vi "Main.vi"() -> ()   [LabVIEW 2020]
doc: "This template is for the Queued Message Handler design pattern.\n\nThe Event Handling Loop generates messages based on user interface actions.\n\nThe Message Handling Loop processes messages generated by the Event Handling Loop, or by other messages. The messages are string values, so new messages can be added easily to the Message Cases case structure in the Message Handling Loop. Each message cluster can also provide an optional value for Message Data, which is a variant that can be converted to whatever message-specific data is required."
uses:
  controls/UI Data.ctl
  support/Message Queue/Enqueue Message (Single).vi
  Global 1.vi
  <vilib>/Utility/error.llb/Error Cluster From Error Code.vi
  <vilib>/ErrorRing/Error Ring.xnode
  support/Message Queue/Message Queue.lvlib
  support/User Event - Stop/User Event - Stop.lvlib
panel:
  in  "Preferences":bool
  in  "Tab Control":enum32{"Main", "New Scenario", "Run Scenario"}(tab)
  in  "New Scenario":bool
  in  "Run Scenario":bool
  in  "Return":bool
  in  "Quit":bool
  in  "Edit Scenario":bool
  in  "Play Button":bool
  in  "Media Stop Button":bool
  out "number (0 to 1)":dbl
  out "Display <Replace Me>":string
  in  "Exit":bool
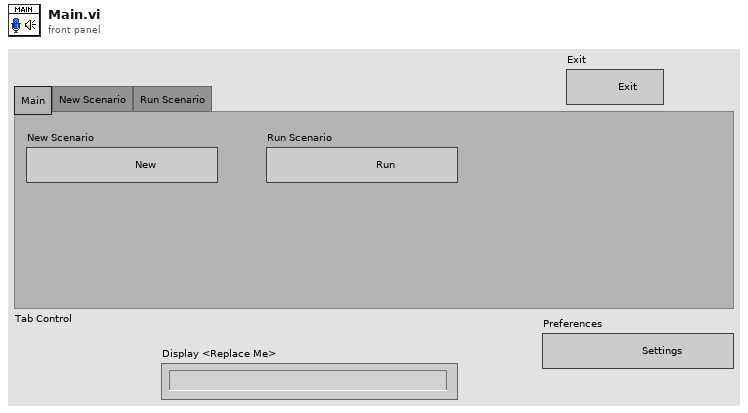
[diagram p1: front panel]
types:
  T1 = typedef "UI Data.ctl" = cluster{"Boolean <Replace Me>":bool, "String <Replace Me>":string, "Numeric <Replace Me>":dbl, "New Scenario Ref":refnum<vi>, "Run Scenario Else Ref":refnum<vi>, "Data Display Ref":refnum<vi>, "Exit Button Ref":refnum<vi>}
  T2 = typedef "Message Queue.lvlib/All Message Queues.ctl" = cluster{"UI":refnum<queue>}
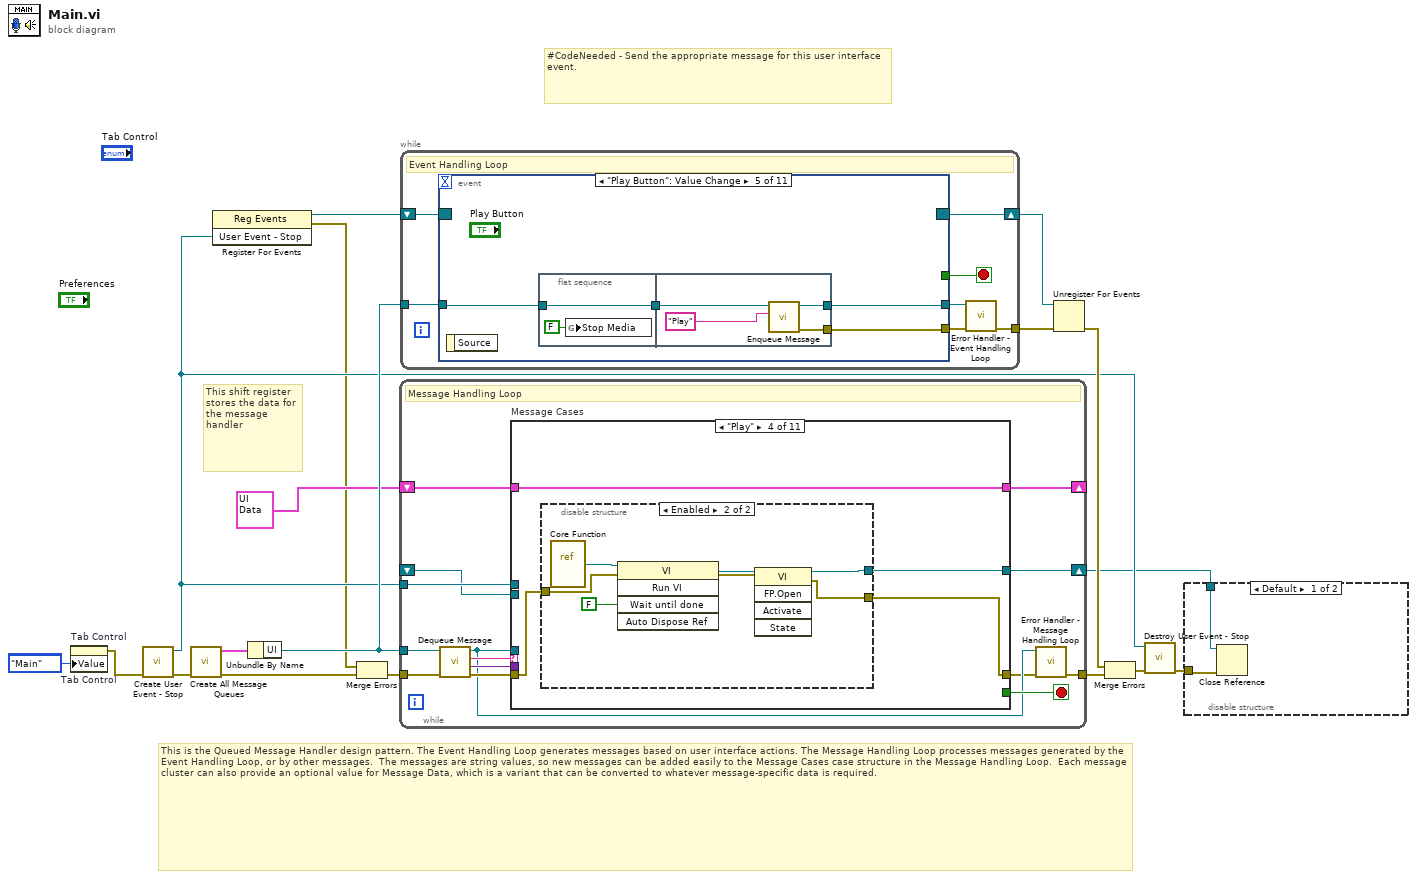
[diagram p0: block diagram]
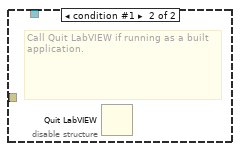
[diagram p2: hidden frame]
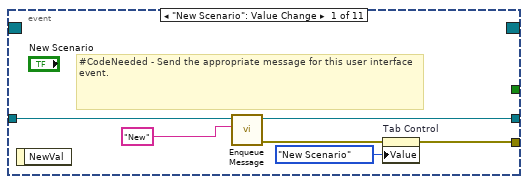
[diagram p3: hidden frame]
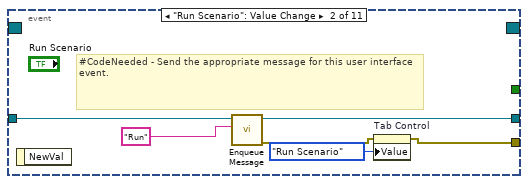
[diagram p4: hidden frame]
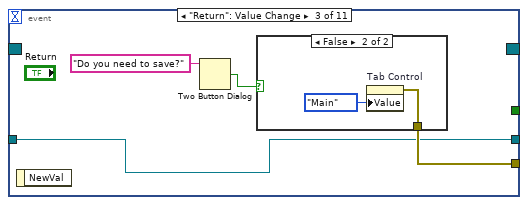
[diagram p5: hidden frame]
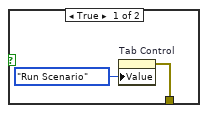
[diagram p6: hidden frame]
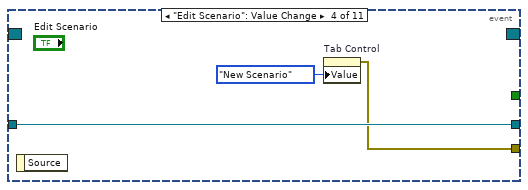
[diagram p7: hidden frame]
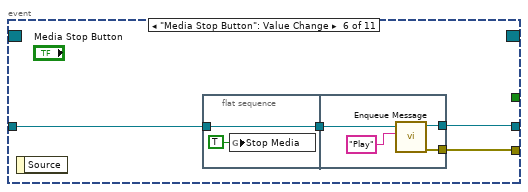
[diagram p8: hidden frame]
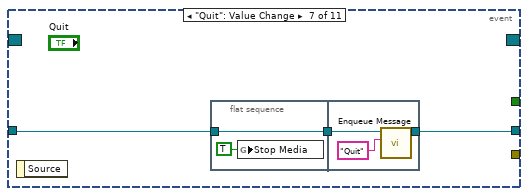
[diagram p9: hidden frame]
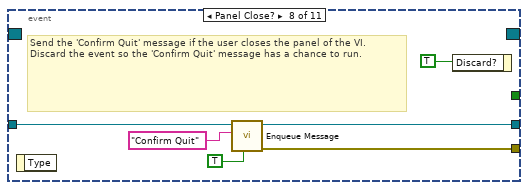
[diagram p10: hidden frame]
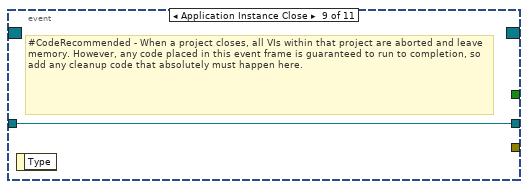
[diagram p11: hidden frame]
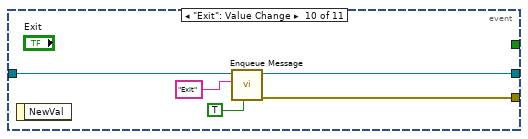
[diagram p12: hidden frame]
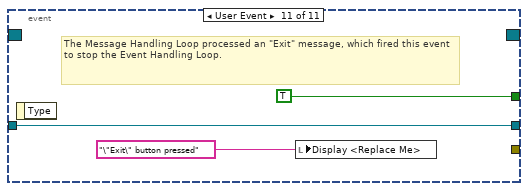
[diagram p13: hidden frame]
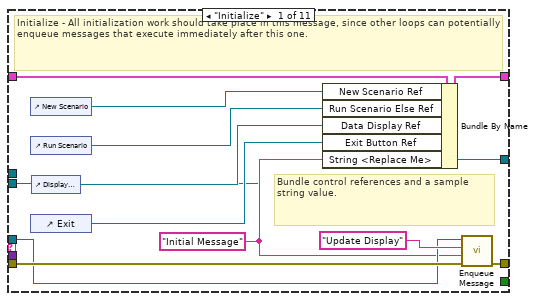
[diagram p14: hidden frame]
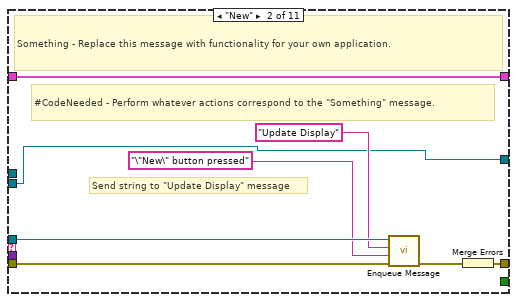
[diagram p15: hidden frame]
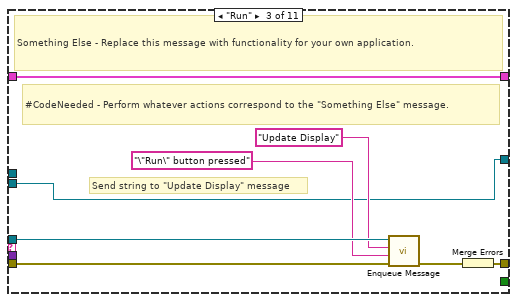
[diagram p16: hidden frame]
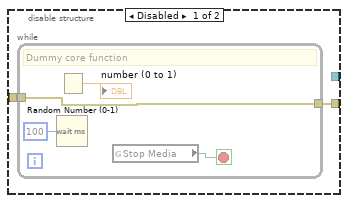
[diagram p17: hidden frame]
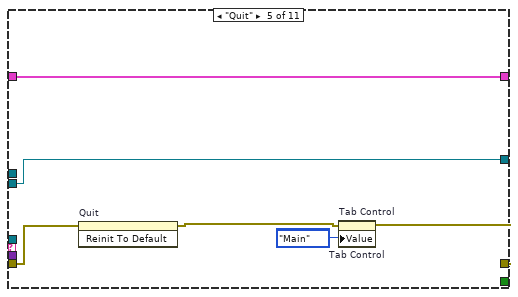
[diagram p18: hidden frame]
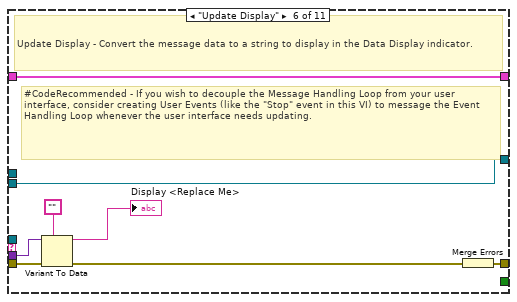
[diagram p19: hidden frame]
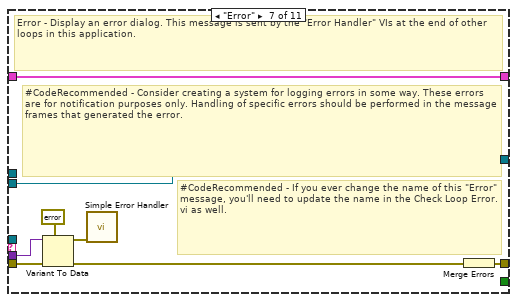
[diagram p20: hidden frame]
diagram:
  # "#CodeNeeded - Send the appropriate message for this user interface event."
  # "This is the Queued Message Handler design pattern. The Event Handling Loop generates messages based on user interface actions. The Message Handling Loop processes messages generated by the Event Handling Loop, or by other messages.  The messages are string values, so new messages can be added easily to the Message Cases case structure in the Message Handling Loop.  Each message cluster can also provide an optional value for Message Data, which is a variant that can be converted to whatever message-specific data is required."
  # "This shift register stores the data for the message handler"
  n1 = property on="Tab Control" class="TabCtl (strict)"("Value"=enum32{"Main", "New Scenario", "Run Scenario"}."Main" ("Tab Control")) -> ()  [unwired: 2 in, 2 out]
  n2 = property on="Tab Control" class="TabCtl (strict)"("Value"=enum32{"Main", "New Scenario", "Run Scenario"}."Main" ("Tab Control")) -> (error out=w3:errorcluster)  [unwired: 2 in, 1 out]
  n3 = call "Create User Event - Stop.vi"("error in (no error)"=w3) -> ("error out"=w15:errorcluster, "User Event - Stop"=w7:refnum<user-event>)  [unwired: 9 in]
  n4 = call "Create All Message Queues.vi"("error in (no error)"=w15) -> ("error out"=w19:errorcluster, "Message Queues out"=w18:T2)  [unwired: 9 in]
  n5 = register-events(w7) -> (reference out=w8:refnum<event-registration>, error out=w5:errorcluster)  [unwired: 2 in]
  n6 = Unbundle By Name(w18) -> ("UI"=w16:refnum<queue>)
  n7 = Merge Errors(w5, w19) -> (w6:errorcluster)
  n8 = while {
    tunnel: w16 -> [w25]
    shift-right: [w32] -> _
    shift-left: T1 {"Boolean <Replace Me>"=FALSE, "String <Replace Me>"="", "Numeric <Replace Me>"=0.0, "New Scenario Ref"=refnum, "Run Scenario Else Ref"=refnum, "Data Display Ref"=refnum, "Exit Button Ref"=refnum} ("Data Cluster") -> [w33]
    tunnel: w7 -> [w30]
    tunnel: w6 -> [w29]
    tunnel: [w23] -> w17
    shift-right: [w21] -> w1
    shift-left: _ -> [w20]
    stop <- w31 stop-if-true
    # "Message Handling Loop"
    n9 = call "Dequeue Message.vi"("error in (no error)"=w29, "Message Queue"=w25) -> ("error out"=w28:errorcluster, "Message Data"=w26:variant, "Message"=w27:string, "dup Message Queue"=w24:refnum<queue>)  [unwired: 6 in]
    n10 = case "Message Cases" shown="\"Play\"" w27 {
      selector: w27 -> [_ _ _ _ _ _ _ _ _ _ w127]
      tunnel: w24 -> [w36 w49 w57 _ _ _ _ w105 _ w125 _]
      tunnel: w28 -> [w44 w51 w59 w64 w81 w91 w101 w109 w113 w119 _]
      tunnel: [w45 w52 w60 w63 w82 w92 w95 w107 w111 w122 w128] -> w22
      tunnel: w33 -> [w43 w53 w61 w65 w85 w93 w100 w108 w112 w124 w129]
      tunnel: [w42 w53 w61 w65 w85 w93 w100 w108 w112 w124 w129] -> w32
      tunnel: [_ _ _ _ _ _ _ _ _ TRUE _] -> w31
      tunnel: w26 -> [_ _ _ _ _ w90 w99 _ _ w116 _]
      tunnel: w30 -> [_ _ _ _ _ _ _ _ _ w121 _]
      tunnel: [w34 w46 w54 w62 w79 w86 w94 w102 w110 w115 w126] -> w21
      tunnel: w20 -> [w34 w46 w54 _ w79 w86 w94 w102 w110 w115 w126]
      frame "Initialize" {
        w35 = "Initial Message" ("Initial Message")
        # "Bundle control references and a sample string value."
        # "Initialize - All initialization work should take place in this message, since other loops can potentially enqueue messages that execute immediately after this one."
        n11 = control-ref of="New Scenario"() -> (w41:refnum<vi>)
        n12 = control-ref of="Run Scenario"() -> (w40:refnum<vi>)
        n13 = control-ref of="Exit"() -> (w38:refnum<vi>)
        n14 = control-ref of="Display <Replace Me>"() -> (w39:refnum<vi>)
        n15 = Bundle By Name(cluster=w43, "New Scenario Ref"=w41, "Run Scenario Else Ref"=w40, "Data Display Ref"=w39, "Exit Button Ref"=w38, "String <Replace Me>"=w35) -> (w42:T1)
        n16 = call-poly "Enqueue Message.vi"("error in (no error)"=w44, "Message Data"=w35, "Message"="Update Display", "Message Queue"=w36) -> ("error out"=w45:errorcluster)  [unwired: 6 in, 1 out]
      }
      frame "New" {
        # "Send string to \"Update Display\" message"
        # "#CodeNeeded - Perform whatever actions correspond to the \"Something\" message."
        # "Something - Replace this message with functionality for your own application."
        n17 = call-poly "Enqueue Message.vi"("error in (no error)"=w51, "Message Data"="\"New\" button pressed" ("\"Do Something\" button pressed"), "Message"="Update Display", "Message Queue"=w49) -> ("error out"=w50:errorcluster)  [unwired: 6 in, 1 out]
        n18 = Merge Errors(w50) -> (w52:errorcluster)
      }
      frame "Run" {
        # "Send string to \"Update Display\" message"
        # "#CodeNeeded - Perform whatever actions correspond to the \"Something Else\" message."
        # "Something Else - Replace this message with functionality for your own application."
        n19 = call-poly "Enqueue Message.vi"("error in (no error)"=w59, "Message Data"="\"Run\" button pressed" ("\"Do Something Else\" button pressed"), "Message"="Update Display", "Message Queue"=w57) -> ("error out"=w58:errorcluster)  [unwired: 6 in, 1 out]
        n20 = Merge Errors(w58) -> (w60:errorcluster)
      }
      frame "Play" {
        n21 = disable-structure shown="Enabled" {
          disable-tunnel: w64 -> [w67 w77]
          disable-tunnel: [w66 w73] -> w63
          disable-tunnel: [_ w72] -> w62
          frame Disabled {
            n22 = while {
              tunnel: w67 -> [w69]
              tunnel: [w69] -> w66
              stop <- w68 stop-if-true
              # "Dummy core function"
              n23 = Wait (ms)(milliseconds to wait=u32 100) -> ()  [unwired: 1 out]
              n24 = Random Number (0-1)() -> (number: 0 to 1=→"number (0 to 1)":dbl)
              n25 = global read "Global 1.vi" "Stop Media"() -> (w68:bool)
            }
          }
          frame Enabled {
            n26 = vi-ref "Core Function.vi"() -> (w78:refnum<vi>)
            n27 = invoke class="VI" method="Run VI"(reference=w78, error in=w77, "Wait until done"=FALSE ("Activate?")) -> (reference out=w75:refnum<vi>, error out=w74:errorcluster)  [unwired: 2 in, 3 out]
            n28 = invoke class="VI" method="FP.Open"(reference=w75, error in=w74) -> (reference out=w72:refnum<vi>, error out=w73:errorcluster)  [unwired: 3 in, 3 out]
          }
        }
      }
      frame "Quit" {
        n29 = invoke on="Quit" class="Bool (strict)" method="Reinit To Default"(error in=w81) -> (error out=w80:errorcluster)  [unwired: 2 in, 2 out]
        n30 = property on="Tab Control" class="TabCtl (strict)"(error in=w80, "Value"=enum32{"Main", "New Scenario", "Run Scenario"}."Main" ("Tab Control")) -> (error out=w82:errorcluster)  [unwired: 1 in, 1 out]
        n31 = property on="Tab Control" class="TabCtl (strict)"("Value"=enum32{"Main", "New Scenario", "Run Scenario"}."Main" ("Tab Control")) -> ()  [unwired: 2 in, 2 out]
      }
      frame "Update Display" {
        # "#CodeRecommended - If you wish to decouple the Message Handling Loop from your user interface, consider creating User Events (like the \"Stop\" event in this VI) to message the Event Handling Loop whenever the user interface needs updating."
        # "Update Display - Convert the message data to a string to display in the Data Display indicator."
        n32 = Variant To Data(error in=w91, type="", Variant=w90) -> (data=→"Display <Replace Me>":string, error out=w88:errorcluster)
        n33 = Merge Errors(w88) -> (w92:errorcluster)
      }
      frame "Error" {
        # "#CodeRecommended - If you ever change the name of this \"Error\" message, you'll need to update the name in the Check Loop Error.vi as well."
        # "#CodeRecommended - Consider creating a system for logging errors in some way. These errors are for notification purposes only. Handling of specific errors should be performed in the message frames that generated the error."
        # "Error - Display an error dialog. This message is sent by the \"Error Handler\" VIs at the end of other loops in this application."
        n34 = Variant To Data(error in=w101, type=errorcluster {"status"=FALSE, "code"=0, "source"=""} ("error constant"), Variant=w99) -> (data=w97:errorcluster, error out=w96:errorcluster)
        n35 = call <vilib>:"Simple Error Handler.vi"("error in (no error)"=w97) -> ()  [unwired: 4 in, 5 out]
        n36 = Merge Errors(w96) -> (w95:errorcluster)
      }
      frame "Confirm Quit" {
        # "#CodeNeeded - If you want to provide an \"Are you sure\" dialog (or some other notification) before the application exits, place that code here. This message is typically sent from a Panel Close? event."
        # "Confirm Quit - Message that can confirm whether or not the user wants to exit the application."
        n37 = call-poly "Enqueue Message.vi"("Priority Message? (F)"=TRUE, "error in (no error)"=w109, "Message"="Exit", "Message Queue"=w105) -> ("error out"=w106:errorcluster)  [unwired: 6 in, 1 out]
        n38 = Merge Errors(w106) -> (w107:errorcluster)
      }
      frame "---Copy This Frame---" {
        # "Duplicate this frame when creating new messages.  Change this comment in the duplicated frame to describe this message."
        n39 = Merge Errors(w113) -> (w111:errorcluster)
      }
      frame "Exit" {
        # "Stop the VI"
        # "Release the message queue reference"
        # "#CodeNeeded - Add any required cleanup code here. Note that if 'Exit' was called as a result of an error, an error dialog will be displayed. Add any custom error handling for an 'Exit' condition here as well."
        # "Exit - Exit the application."
        n40 = Variant To Data(type=errorcluster {"status"=FALSE, "code"=0, "source"=""} ("error constant"), Variant=w116) -> (data=w117:errorcluster)  [unwired: 1 in, 1 out]
        n41 = call <vilib>:"Simple Error Handler.vi"("error in (no error)"=w117) -> ()  [unwired: 4 in, 5 out]
        n42 = call "Fire User Event - Stop.vi"("User Event - Stop"=w121) -> ("error out"=w120:errorcluster)  [unwired: 10 in]
        n43 = Release Queue(queue=w125, error in (no error)=w119) -> (error out=w114:errorcluster)  [unwired: 1 in, 2 out]
        n44 = Merge Errors(w120, w114) -> (w122:errorcluster)
      }
      frame Default {
        # "'Default' case only runs if there is a message that isn't defined in any of the other cases.  Output a programming error."
        n45 = xnode "Error Ring"("parameter 0"=w127) -> ("error out"=w128:errorcluster)
      }
    }
    n46 = call "Error Handler - Message Handling Loop.vi"("error in (no error)"=w22, "Message Queue"=w24) -> ("dup error in"=w23:errorcluster)  [unwired: 8 in, 1 out]
  }
  n47 = while {
    tunnel: w16 -> [w143]
    shift-right: [w141] -> w12
    shift-left: w8 -> [w142]
    tunnel: [w137] -> w9
    stop <- w139 stop-if-true
    # "Event Handling Loop"
    n48 = event shown="[4] \"Play Button\": Value Change" {
      selector: w142 -> [_ _ _ _ _ _ _ _ _ _ _]
      dyn-events: [_ _ _ _ _ _ _ _ _ _ _] -> w141
      timeout: _ -> [_ _ _ _ _ _ _ _ _ _ _]
      tunnel: [_ _ _ _ _ _ _ _ _ _ TRUE ("Discard?")] -> w139
      tunnel: w143 -> [w149 w155 w158 w166 w168 w180 w188 w199 w201 w206 w209]
      tunnel: [w146 w151 w159 w164 w169 w177 _ w198 _ w205 _] -> w140
      tunnel: [w148 w154 w158 w166 w170 w178 w189 w197 w201 w204 w209] -> w138
      event "New Scenario": Value Change {
        # "#CodeNeeded - Send the appropriate message for this user interface event."
        n49 = event-data() -> ()  [unwired: 1 in, 1 out]
        n50 = call-poly "Enqueue Message.vi"("Message"="New", "Message Queue"=w149) -> ("error out"=w145:errorcluster, "dup Message Queue"=w148:refnum<queue>)  [unwired: 8 in]
        n51 = property on="Tab Control" class="TabCtl (strict)"(error in=w145, "Value"=enum32{"Main", "New Scenario", "Run Scenario"}."New Scenario" ("Tab Control")) -> (error out=w146:errorcluster)  [unwired: 1 in, 1 out]
      }
      event "Run Scenario": Value Change {
        # "#CodeNeeded - Send the appropriate message for this user interface event."
        n52 = event-data() -> ()  [unwired: 1 in, 1 out]
        n53 = call-poly "Enqueue Message.vi"("Message"="Run", "Message Queue"=w155) -> ("error out"=w152:errorcluster, "dup Message Queue"=w154:refnum<queue>)  [unwired: 8 in]
        n54 = property on="Tab Control" class="TabCtl (strict)"(error in=w152, "Value"=enum32{"Main", "New Scenario", "Run Scenario"}."Run Scenario" ("Tab Control")) -> (error out=w151:errorcluster)  [unwired: 1 in, 1 out]
      }
      event "Return": Value Change {
        n55 = event-data() -> ()  [unwired: 1 in, 1 out]
        n56 = Two Button Dialog(message="Do you need to save?") -> (T button?=w157:bool)  [unwired: 2 in]
        n57 = case shown="False" w157 {
          tunnel: [w161 w163] -> w159
          frame True {
            n58 = property on="Tab Control" class="TabCtl (strict)"("Value"=enum32{"Main", "New Scenario", "Run Scenario"}."Run Scenario" ("Tab Control")) -> (error out=w161:errorcluster)  [unwired: 2 in, 1 out]
          }
          frame False {
            n59 = property on="Tab Control" class="TabCtl (strict)"("Value"=enum32{"Main", "New Scenario", "Run Scenario"}."Main" ("Tab Control")) -> (error out=w163:errorcluster)  [unwired: 2 in, 1 out]
          }
        }
      }
      event "Edit Scenario": Value Change {
        n60 = event-data() -> ()  [unwired: 1 in, 1 out]
        n61 = property on="Tab Control" class="TabCtl (strict)"("Value"=enum32{"Main", "New Scenario", "Run Scenario"}."New Scenario" ("Tab Control")) -> (error out=w164:errorcluster)  [unwired: 2 in, 1 out]
      }
      event "Play Button": Value Change {
        n62 = event-data() -> ()  [unwired: 1 in, 1 out]
        n63 = flat-sequence {
          tunnel: w168 -> [w172]
          tunnel: [w172] -> w167
          tunnel: [w175] -> w170
          tunnel: [w174] -> w169
          tunnel: w167 -> [w173]
          frame #0 {
            n64 = global write "Global 1.vi" "Stop Media"(FALSE ("Stop Media")) -> ()
          }
          frame #1 {
            n65 = call-poly "Enqueue Message.vi"("Message"="Play", "Message Queue"=w173) -> ("error out"=w174:errorcluster, "dup Message Queue"=w175:refnum<queue>)  [unwired: 8 in]
          }
        }
      }
      event "Media Stop Button": Value Change {
        n66 = event-data() -> ()  [unwired: 1 in, 1 out]
        n67 = flat-sequence {
          tunnel: w180 -> [w181]
          tunnel: [w181] -> w179
          tunnel: w179 -> [w185]
          tunnel: [w184] -> w178
          tunnel: [w183] -> w177
          frame #0 {
            n68 = global write "Global 1.vi" "Stop Media"(TRUE ("Stop Media")) -> ()
          }
          frame #1 {
            n69 = call-poly "Enqueue Message.vi"("Message"="Play", "Message Queue"=w185) -> ("error out"=w183:errorcluster, "dup Message Queue"=w184:refnum<queue>)  [unwired: 8 in]
          }
        }
      }
      event "Quit": Value Change {
        n70 = event-data() -> ()  [unwired: 1 in, 1 out]
        n71 = flat-sequence {
          tunnel: w188 -> [w191]
          tunnel: [w191] -> w187
          tunnel: [w193] -> w189
          tunnel: w187 -> [w192]
          frame #0 {
            n72 = global write "Global 1.vi" "Stop Media"(TRUE ("Stop Media")) -> ()
          }
          frame #1 {
            n73 = call-poly "Enqueue Message.vi"("Message"="Quit", "Message Queue"=w192) -> ("dup Message Queue"=w193:refnum<queue>)  [unwired: 8 in, 1 out]
          }
        }
      }
      event Panel Close? {
        # "Send the 'Confirm Quit' message if the user closes the panel of the VI. Discard the event so the 'Confirm Quit' message has a chance to run."
        n74 = event-data() -> ()  [unwired: 1 in, 1 out]
        n75 = call-poly "Enqueue Message.vi"("Priority Message? (F)"=TRUE, "Message"="Confirm Quit", "Message Queue"=w199) -> ("error out"=w198:errorcluster, "dup Message Queue"=w197:refnum<queue>)  [unwired: 7 in]
        n76 = event-data("Discard?"=TRUE) -> ()  [unwired: 1 in, 1 out]
      }
      event Application Instance Close {
        # "#CodeRecommended - When a project closes, all VIs within that project are aborted and leave memory. However, any code placed in this event frame is guaranteed to run to completion, so add any cleanup code that absolutely must happen here."
        n77 = event-data() -> ()  [unwired: 1 in, 1 out]
      }
      event "Exit": Value Change {
        n78 = event-data() -> ()  [unwired: 1 in, 1 out]
        n79 = call-poly "Enqueue Message.vi"("Priority Message? (F)"=TRUE, "Message"="Exit", "Message Queue"=w206) -> ("error out"=w205:errorcluster, "dup Message Queue"=w204:refnum<queue>)  [unwired: 7 in]
      }
      event User Event {
        # "The Message Handling Loop processed an \"Exit\" message, which fired this event to stop the Event Handling Loop."
        n80 = event-data() -> ()  [unwired: 1 in, 1 out]
        n81 = local write "Display <Replace Me>"("\"Exit\" button pressed" ("VI Stopped")) -> ()
      }
    }
    n82 = call "Error Handler - Event Handling Loop.vi"("error in (no error)"=w140, "Message Queue"=w138) -> ("dup error in"=w137:errorcluster)  [unwired: 8 in, 1 out]
  }
  n83 = Unregister For Events(event registration refnum=w12, error in=w9) -> (error out=w13:errorcluster)
  n84 = Merge Errors(w13, w17) -> (w14:errorcluster)
  n85 = call "Destroy User Event - Stop.vi"("error in (no error)"=w14, "User Event - Stop"=w7) -> ("error out"=w10:errorcluster)  [unwired: 9 in]
  n86 = disable-structure shown="Default" {
    disable-tunnel: w10 -> [w211 _]
    disable-tunnel: w1 -> [w210 _]
    frame condition #0 (active) {
      n87 = Close Reference(reference=w210, error in (no error)=w211) -> ()  [unwired: 1 out]
    }
    frame condition #1 {
      # "Call Quit LabVIEW if running as a built application."
      n88 = Quit LabVIEW() -> ()  [unwired: 1 in]
    }
  }
